vi "savecluster_V0.01.vi"(1 "selected path":path, 2 "Datenspeicher 3":refnum<vi>) -> ()   [LabVIEW 2014]
uses:
  <vilib>/Utility/xml.llb/Write to XML File(string).vi
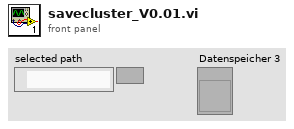
[diagram p1: front panel]
types:
  T1 = cluster{"Fahrzeugdaten":string, "date/time string":string, "Rolle [Inkr/U]":u16, "Rollenumfang [m]":dbl, "Rollenträgheit [kgm²]":dbl, "Zündung [Imp/U]":dbl, "Getriebe [1:]":dbl, "Reifenumfang [m] ":dbl, "element":dbl, "Gl. Mittelwert":u8, "Differenzenquotient":u8, "Polynom":u8, "element":dbl, "element":dbl, "Lufttemperatur [°C]":dbl, "Luftfeuchtigkeit [%]":dbl, "Luftdruck [mbar]":dbl, dbl[], dbl[], "Best Polynomial Fit":dbl[], dbl[], "Übersetzung ermitteln aus":u8, "[s]":dbl, "nmin [1/min]":dbl, "nmax [1/min]":dbl, "n vom Gas [1/min]":dbl, dbl[], i32[], "Boolesch":bool, "Serielle Schnittstelle":refnum<visa-resource-name>, "nKuWe/nRolle 2":dbl}
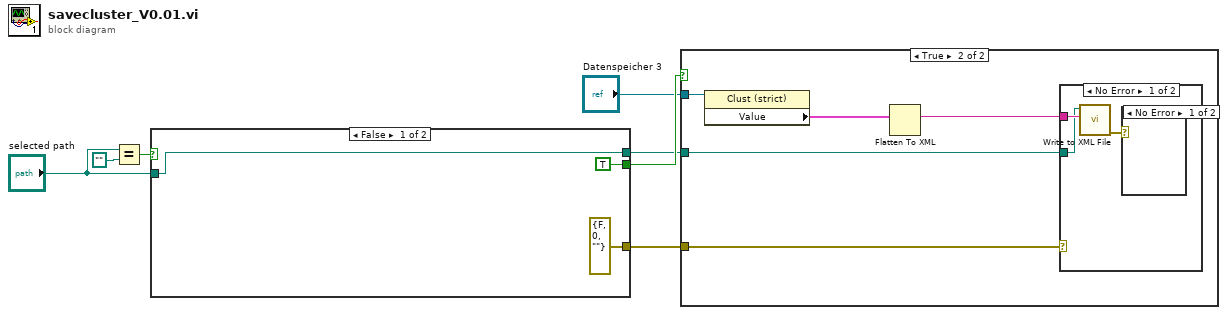
[diagram p0: block diagram]
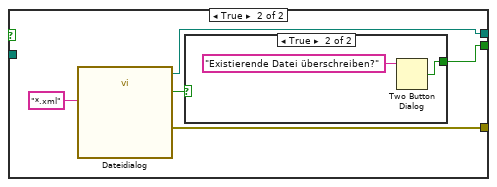
[diagram p2: hidden frame]
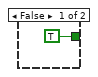
[diagram p3: hidden frame]
diagram:
  n1 = Equal?(x="selected path", y=path "") -> (x = y?=w3:bool)
  n2 = case shown="False" w3 {
    tunnel: [TRUE ("T button?") w15] -> w7
    tunnel: [errorcluster {"status"=FALSE, "code"=0, "source"=""} ("error out") w13] -> w6
    tunnel: [w9 w12] -> w5
    tunnel: "selected path" -> [w9 _]
    frame False {
    }
    frame True {
      n3 = call "Dateidialog"("pattern (all files)"="*.xml") -> ("selected path"=w12:path, "exists"=w14:bool, "error out"=w13:errorcluster)  [unwired: 11 in, 1 out]
      n4 = case shown="True" w14 {
        tunnel: [TRUE ("T button?") w17] -> w15
        frame False {
        }
        frame True {
          n5 = Two Button Dialog(message="Existierende Datei überschreiben?" ("Nachricht")) -> (T button?=w17:bool)  [unwired: 2 in]
        }
      }
    }
  }
  n6 = case shown="True" w7 {
    tunnel: w5 -> [_ w23]
    tunnel: w6 -> [_ w22]
    tunnel: "Datenspeicher 3" -> [_ w20]
    frame False {
    }
    frame True {
      n7 = property class="Clust (strict)"(reference=w20) -> ("Value"=w19:T1)  [unwired: 1 in, 2 out]
      n8 = Flatten To XML(anything=w19) -> (xml string=w21:string)
      n9 = case shown="No Error" w22 {
        tunnel: w21 -> [w26 _]
        tunnel: w23 -> [w24 _]
        frame No Error {
          n10 = call-poly <vilib>:"Write to XML File.vi"("XML Input"=w26, "XML File Path"=w24) -> ("error out"=w25:errorcluster)  [unwired: 7 in, 2 out]
          n11 = case shown="No Error" w25 {
            frame No Error {
            }
            frame Error {
            }
          }
        }
        frame Error {
        }
      }
    }
  }
